vi "ParceDataLoop.vi"(8 "error in (no error)":errorcluster, 11 "SV_Publisher in":refnum<class "SV_Publisher.lvclass">) -> (0 "error out":errorcluster)   [LabVIEW 2019, in "SV_Publisher.lvclass"]
uses:
  SV_Publisher.lvclass
  SV_Publisher.lvclass/SV_Publisher.ctl
  SV_Wrap/SharedVariableWrapper.lvclass/SharedVariableWrapper.ctl
  913bd84b-c2ba-4b0c-b6ec-f85e1833216a.vi
  913bd84b-c2ba-4b0c-b6ec-f85e1833216a.vi/cff770ba-d631-41a9-83c6-8504435118aa.vi
  SV_Wrap/Write Var Info.vi
  SV_Wrap/Read Var Info.vi
  SV_Wrap/Read connection str.vi
  <userlib>/_OpenG.lib/time/time.llb/Tick Count (ms)__ogtk.vi
  3bf26c70-06b2-41b8-8743-e05c4733868f.vi
panel:
  out "Data dub":variant
  out "name dub":string
  out "x+1":i32
  out "SET SV Error 2":errorcluster
  out "SET SV Error":errorcluster
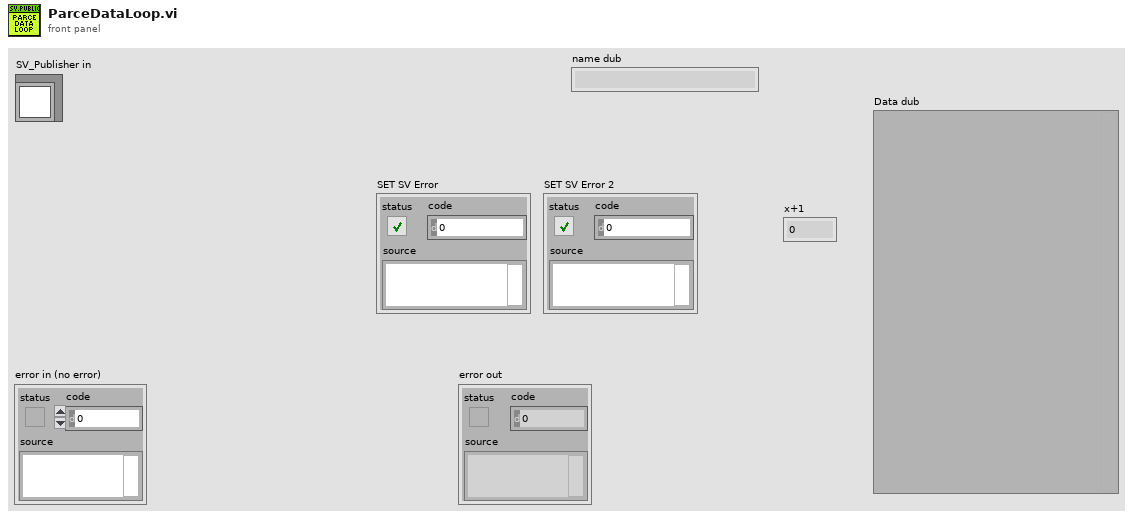
[diagram p1: front panel]
types:
  T1 = typedef "SV_Publisher.lvclass/Data.ctl" = cluster{"Name":string, "Value":variant}
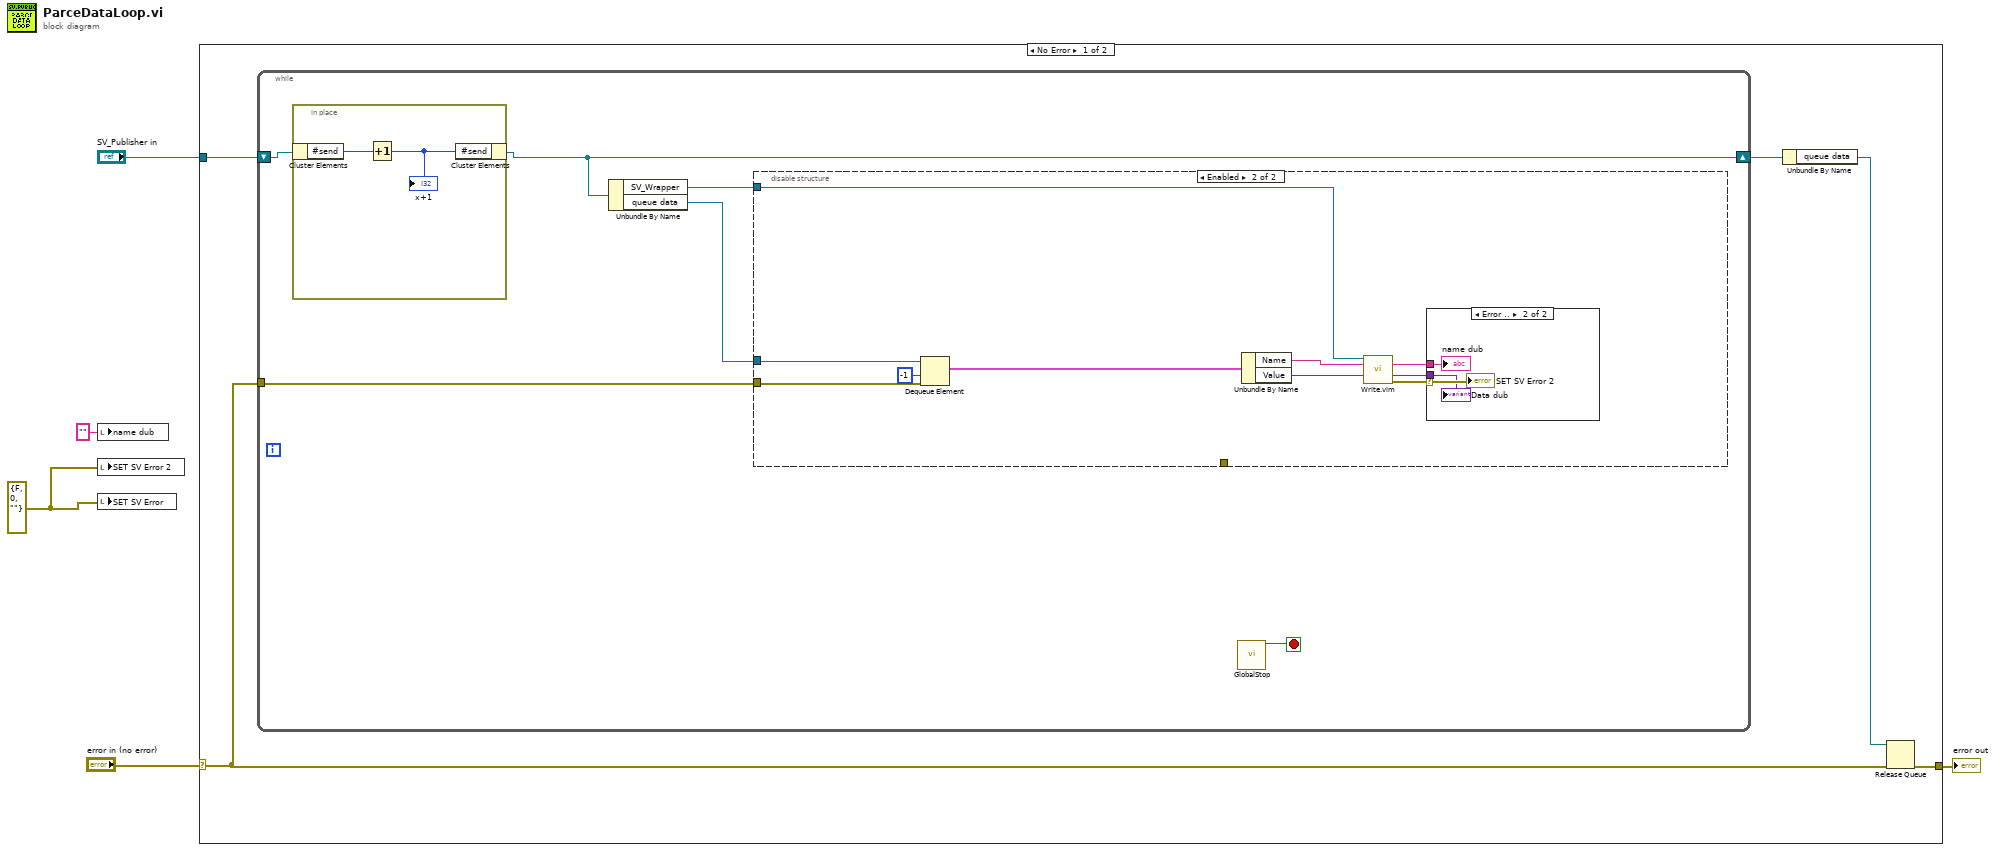
[diagram p0: block diagram]
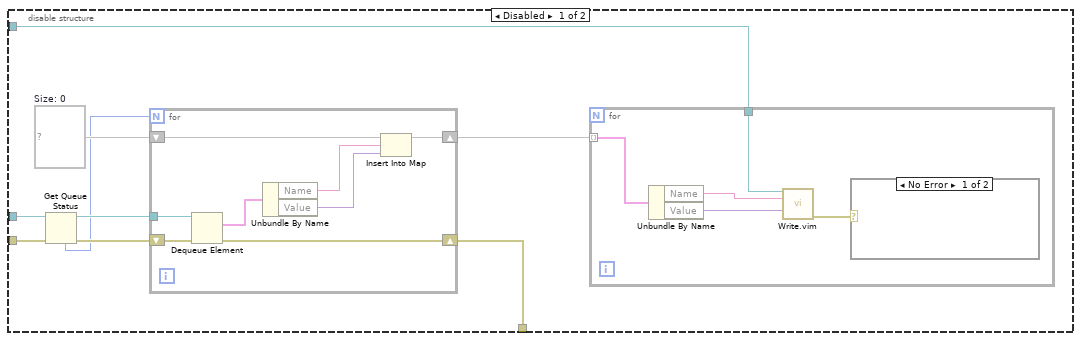
[diagram p2: hidden frame]
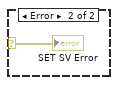
[diagram p3: hidden frame]
diagram:
  w1 = errorcluster {"status"=FALSE, "code"=0, "source"=""} ("SET SV Error")
  n1 = local write "name dub"("" ("name dub")) -> ()
  n2 = local write "SET SV Error 2"(w1) -> ()
  n3 = local write "SET SV Error"(w1) -> ()
  n4 = case shown="No Error" "error in (no error)" {
    selector: "error in (no error)" -> [w7 w55]
    tunnel: [w6 w55] -> w4
    tunnel: "SV_Publisher in" -> [w10 _]
    frame No Error {
      n5 = while {
        shift-right: [w12] -> w9
        shift-left: w10 -> [w13]
        tunnel: w7 -> [w14]
        stop <- w11 stop-if-true
        n6 = in-place {
          n7 = in-place-cluster #1(w13) -> ("#send"=w18:i32)
          n8 = Increment(x=w18) -> (x+1=w17:i32)
          "x+1" <- w17
          n9 = in-place-cluster #1("#send"=w17) -> (w12:refnum<class "SV_Publisher.lvclass">)
        }
        n10 = Unbundle By Name(w12) -> ("SV_Wrapper"=w16:refnum<class "SharedVariableWrapper.lvclass">, "queue data"=w15:refnum<queue>)
        n11 = disable-structure shown="Enabled" {
          disable-tunnel: w16 -> [w27 w51]
          disable-tunnel: w15 -> [w26 w50]
          disable-tunnel: w14 -> [w25 w49]
          disable-tunnel: [w22 _] -> _
          frame Disabled {
            w21 = map{string, variant} {}  # Size: 0
            n12 = Get Queue Status(queue=w26, error in (no error)=w25) -> (queue out=w24:refnum<queue>, error out=w23:errorcluster, # elements in queue=w19:i32)  [unwired: 1 in, 5 out]
            n13 = for {
              N: w19 -> [_]
              tunnel: w24 -> [w40]
              shift-right: [w38] -> w22
              shift-left: w23 -> [w39]
              shift-right: [w35] -> w20
              shift-left: w21 -> [w34]
              n14 = Dequeue Element(queue=w40, error in (no error)=w39) -> (element=w41:T1, error out=w38:errorcluster)  [unwired: 1 in, 2 out]
              n15 = Unbundle By Name(w41) -> ("Name"=w37:string, "Value"=w36:variant)
              n16 = Insert Into Map(map in=w34, key=w37, value=w36) -> (map out=w35:map{string, variant})  [unwired: 2 out]
            }
            n17 = for {
              tunnel: w27 -> [w32]
              tunnel: w20 -> [w30] mode=indexing
              n18 = Unbundle By Name(w30) -> ("Name"=w29:string, "Value"=w28:variant)
              n19 = call "Write.vim"("SharedVariableWrapper in"=w32, "name"=w29, "Data"=w28) -> ("error out"=w31:errorcluster)  [unwired: 6 in, 6 out]
              n20 = case shown="No Error" w31 {
                selector: w31 -> [_ w33]
                frame No Error {
                }
                frame Error {
                  "SET SV Error" <- w33
                }
              }
            }
          }
          frame Enabled {
            n21 = Dequeue Element(queue=w50, timeout in ms (-1)=-1, error in (no error)=w49) -> (element=w45:T1)  [unwired: 3 out]
            n22 = Unbundle By Name(w45) -> ("Name"=w47:string, "Value"=w46:variant)
            n23 = call "Write.vim"("SharedVariableWrapper in"=w51, "name"=w47, "Data"=w46) -> ("name dub"=w43:string, "Data dub"=w42:variant, "error out"=w48:errorcluster)  [unwired: 6 in, 4 out]
            n24 = case shown="Error .." w48 {
              selector: w48 -> [_ w54]
              tunnel: w43 -> [_ w53]
              tunnel: w42 -> [_ w52]
              frame No Error {
              }
              frame Error {
                "SET SV Error 2" <- w54
                "name dub" <- w53
                "Data dub" <- w52
              }
            }
          }
        }
        n25 = call "GlobalStop.vi"() -> ("Stop"=w11:bool)  [unwired: 15 in]
      }
      n26 = Unbundle By Name(w9) -> ("queue data"=w8:refnum<queue>)
      n27 = Release Queue(queue=w8, error in (no error)=w7) -> (error out=w6:errorcluster)  [unwired: 1 in, 2 out]
    }
    frame Error {
    }
  }
  "error out" <- w4
